vi "Get Size.vi"(8 "error in (no error)":errorcluster, 11 "CIPC Reference":u64) -> (0 "error out":errorcluster, 3 "Size Info":T1)   [LabVIEW 2021, in "CIF_NI_CIPC.lvlib"]
uses:
  CIF_NI_CIPC.lvlib
  TypeDefs/Info Size.ctl
  libnicipc.dll
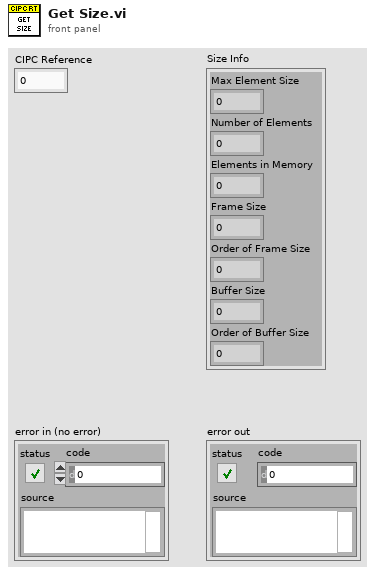
[diagram p1: front panel]
types:
  T1 = typedef "CIF_NI_CIPC.lvlib/Info Size.ctl" = cluster{"Max Element Size":u32, "Number of Elements":u32, "Elements in Memory":u32, "Frame Size":u32, "Order of Frame Size":u32, "Buffer Size":u32, "Order of Buffer Size":u32}
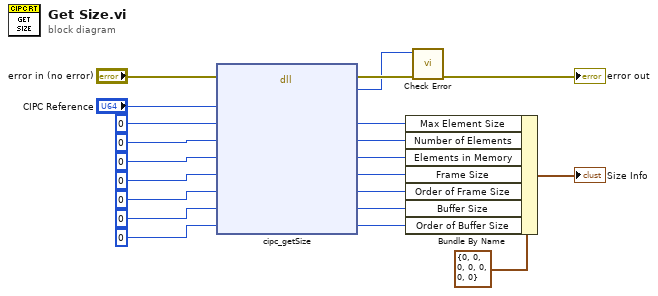
[diagram p0: block diagram]
diagram:
  n1 = dll-call lib="libnicipc.*" fn="cipc_getSize"(error in="error in (no error)", "cipc_buffer_ref"="CIPC Reference", "el_size"=u32 0 ("head"), "nr_elements"=u32 0 ("frame_size"), "nr_elements_in_memory"=u32 0 ("frame_size"), "frame_size"=u32 0, "order_of_frame_size"=u32 0, "buffer_size"=u32 0, "order_of_buffer_size"=u32 0) -> (error out=w15:errorcluster, "return type"=w14:i32, "el_size"=w11:u32, "nr_elements"=w10:u32, "nr_elements_in_memory"=w9:u32, "frame_size"=w8:u32, "order_of_frame_size"=w7:u32, "buffer_size"=w6:u32, "order_of_buffer_size"=w5:u32)  [unwired: 3 in, 1 out]
  n2 = Bundle By Name(cluster=T1 {"Max Element Size"=0, "Number of Elements"=0, "Elements in Memory"=0, "Frame Size"=0, "Order of Frame Size"=0, "Buffer Size"=0, "Order of Buffer Size"=0}, "Max Element Size"=w11, "Number of Elements"=w10, "Elements in Memory"=w9, "Frame Size"=w8, "Order of Frame Size"=w7, "Buffer Size"=w6, "Order of Buffer Size"=w5) -> (→"Size Info":T1)
  n3 = call "Check Error.vi"("error in (no error)"=w15, "Error Code"=w14) -> ("error out"=→"error out":errorcluster)  [unwired: 9 in]
